vi "CloseAdaptorr00.vi"   [LabVIEW 2011]
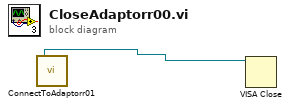
[diagram p0: block diagram]
diagram:
  n1 = call "ConnectToAdaptorr01.vi"() -> ("VISA resource name out"=w1:refnum<visa-resource-name>)  [unwired: 1 in, 1 out]
  n2 = VISA Close(VISA resource name=w1) -> ()  [unwired: 1 in, 1 out]
